vi "Button Handler.vi"(8 "error in (no error)":errorcluster, 11 "Buttons":bool[](array[boolean])) -> (0 "error out":errorcluster)   [LabVIEW 2015]
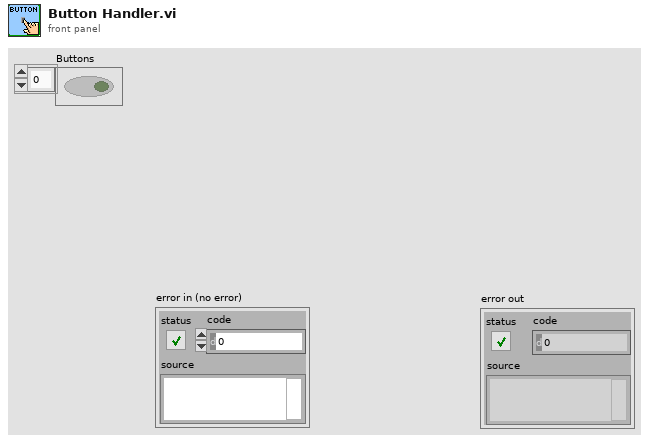
[diagram p1: front panel]
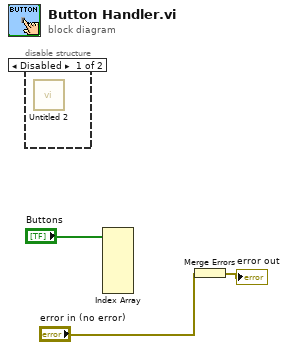
[diagram p0: block diagram]
diagram:
  n1 = disable-structure shown="Disabled" {
    frame Disabled {
      n2 = call "Untitled 2.vi"() -> ()  [unwired: 11 in, 1 out]
    }
    frame Enabled {
    }
  }
  n3 = Index Array(array="Buttons") -> ()  [unwired: 6 in, 6 out]
  n4 = Merge Errors("error in (no error)") -> (→"error out":errorcluster)
